vi "ACM RFPM Calibration Verify .vi"() -> ()   [LabVIEW 2023, in "ACM Visa Driver.lvlib"]
uses:
  ACM Visa Driver.lvlib
  API/Controls/ACM Paths.ctl
  API/Controls/ACM Switch States.ctl
  HFNetworkAnalysis/Controls/Unit.ctl
  HFNetworkAnalysis/Controls/Quantity.ctl
  <instrlib>/niRFPM/niRFPM.llb/NI-RFPM Fetch S-Parameter Measurements Complex.vi
  HFNetworkAnalysis/Support VIs/Convert Unit (DBL Array).vi
  HFNetworkAnalysis/NI_HFNetworkAnalysis.lvlib
panel:
  in  "Tab Control":enum32{"Magnitude", "Phase"}(tab)
  out "Magnitude":T1(array[cluster])=[[{"XY Graph"=[{"frequency"=array[531 elements], "yi"=array[531 elements]}, {"frequency"=array[531 elements], "yi"=array[531 elements]}], "String"="S11"}, {"XY Graph"=[{"frequency"=array[531 elements], "yi"=array[531 elements]}, {"frequency"=array[531 elements], "yi"=array[531 elements]}], "String"="S12"}], [{"XY Graph"=[{"frequency"=array[531 elements], "yi"=array[531 elements]}, {"frequency"=array[531 elements], "yi"=array[531 elements]}], "String"="S21"}, {"XY Graph"=[{"frequency"=array[531 elements], "yi"=array[531 elements]}, {"frequency"=array[531 elements], "yi"=array[531 elements]}], "String"="S22"}]]
  out "Phase":T1(array[cluster])=[[{"XY Graph"=[{"frequency"=array[531 elements], "yi"=array[531 elements]}, {"frequency"=array[531 elements], "yi"=array[531 elements]}], "String"="S11"}, {"XY Graph"=[{"frequency"=array[531 elements], "yi"=array[531 elements]}, {"frequency"=array[531 elements], "yi"=array[531 elements]}], "String"="S12"}], [{"XY Graph"=[{"frequency"=array[531 elements], "yi"=array[531 elements]}, {"frequency"=array[531 elements], "yi"=array[531 elements]}], "String"="S21"}, {"XY Graph"=[{"frequency"=array[531 elements], "yi"=array[531 elements]}, {"frequency"=array[531 elements], "yi"=array[531 elements]}], "String"="S22"}]]
  in  "ACM Ports":T2[](array[typedef])=["A", "B"]
  in  "ACM resource name":refnum<visa-resource-name>="USB0::0x2226::0x000F::00000000::INSTR"
  in  "Sweep Setting Name":string="vectorSweep"
  in  "RFPM Ports":string[](array[string])=["port25", "port27"]
  in  "Calibration Storage File Path":path=path "C:/jenkins/workspace/InstallRunCentaurus1910@2/Sales/Semi/projects/RF Calibration/CM ACM VISA Driver/docs/Vulcan_Msmt_VBF-4440/ACM4509_TXecal_RXecal/NI5534_ACM4509_TXecal_RXecal_LowPwr_100HzRBW.tdms"
  out "error out":errorcluster {"code" format="%.0x"}
  in  "Switch":refnum<k15>="VST0" caption="logical name (\"SampleSwitch\")"
  in  "VST":refnum<k15>="VST0"
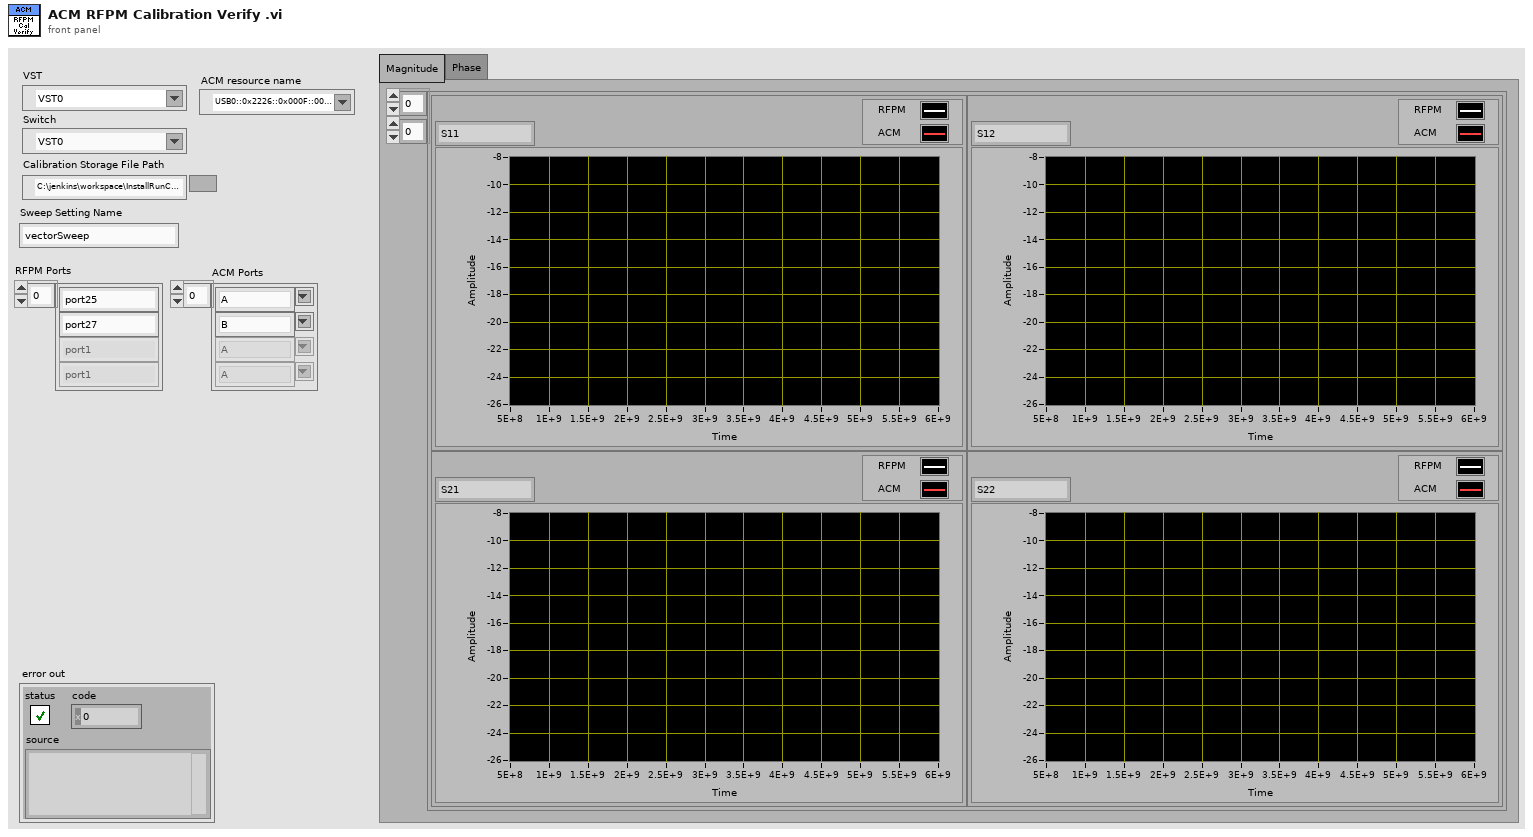
[diagram p1: front panel]
types:
  T1 = cluster{"XY Graph":cluster{"frequency":dbl[], "yi":dbl[]}[], "String":string}[][]
  T2 = typedef "ACM Visa Driver.lvlib/ACM Paths.ctl" = string
  T3 = typedef "ACM Visa Driver.lvlib/ACM Switch States.ctl" = string
  T4 = typedef "NI_HFNetworkAnalysis.lvlib/Unit.ctl" = enum16{"No", "s", "Hz", "V", "A", "Ohm", "W", "dB", "dBV", "dBA", "dBm", "percent", "rad", "deg"}
  T5 = typedef "NI_HFNetworkAnalysis.lvlib/Quantity.ctl" = enum16{"Undefined", "V", "I", "A", "B", "P", "Z", "PowerRatio", "Gamma", "Index"}
  T6 = cluster{"frequency":dbl[], "Converted Data":dbl[]}
  T7 = cluster{"frequency":dbl[], "Converted Data":dbl[]}[]
  T8 = cluster{cluster{"frequency":dbl[], "Converted Data":dbl[]}[], string}
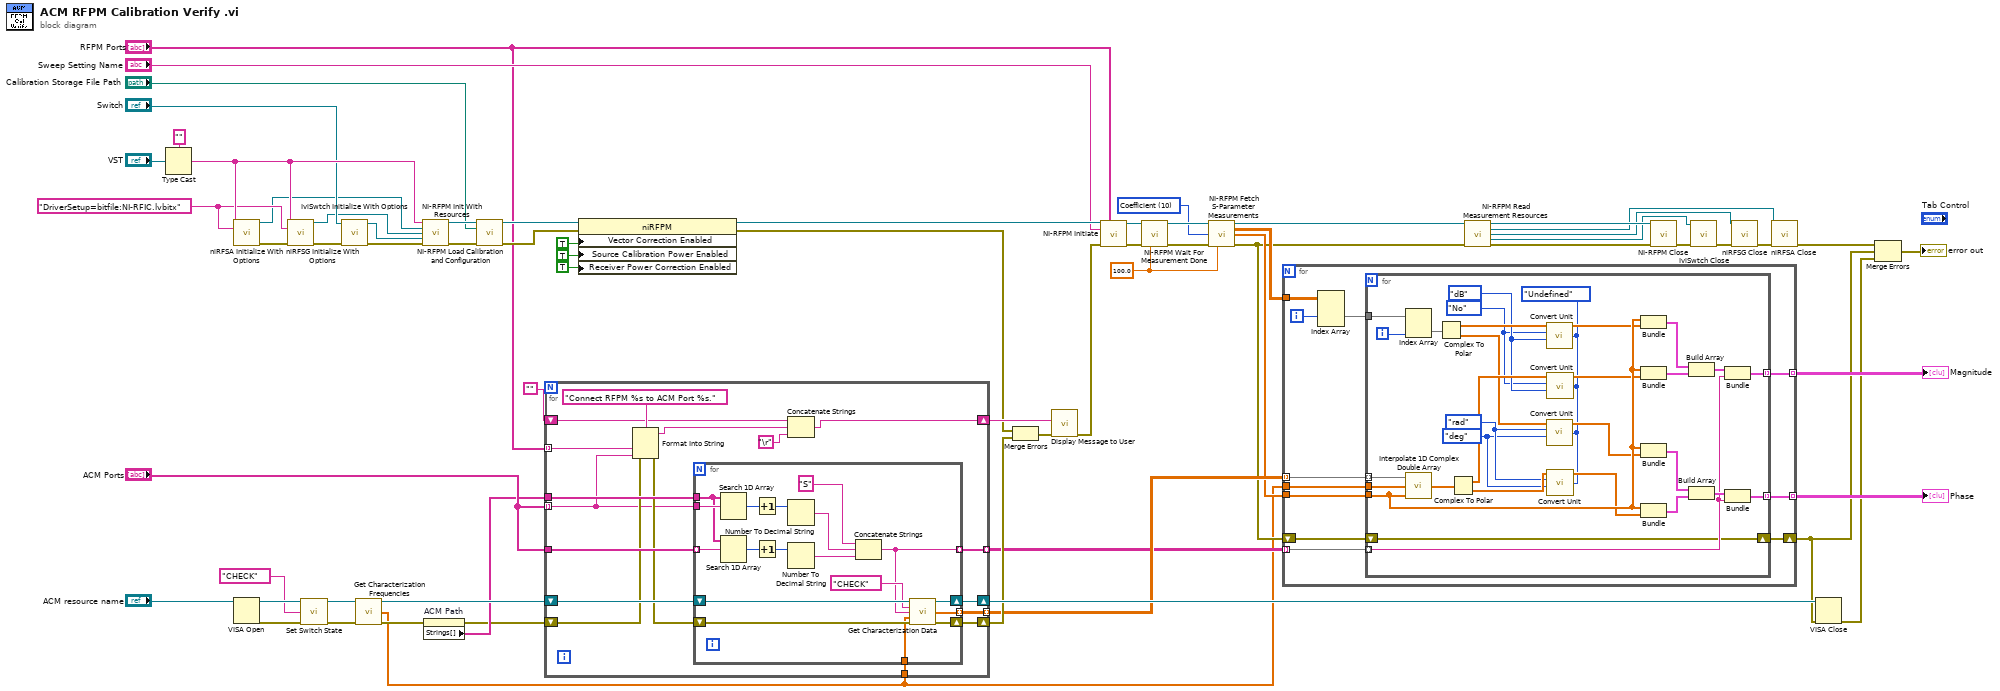
[diagram p0: block diagram]
diagram:
  w54 = 100.0 ("Timeout")
  w53 = 10 items=["Coefficient"=10] ("format")
  w64 = "DriverSetup=bitfile:NI-RFIC.lvbitx"
  n1 = Type Cast(type="", x="VST") -> (*(type *) &x=w65:string)
  n2 = call <instrlib>:"niRFSA Initialize With Options.vi"("resource name"=w65, "option string"=w64) -> ("instrument handle out"=w40:refnum<k15>, "error out"=w44:errorcluster)  [unwired: 12 in]
  n3 = VISA Open(VISA resource name="ACM resource name") -> (VISA resource name=w28:refnum<visa-resource-name>, error out=w30:errorcluster)  [unwired: 4 in]
  n4 = call <instrlib>:"niRFSG Initialize With Options.vi"("resource name"=w65, "option string"=w64, "error in"=w44) -> ("instrument handle"=w41:refnum<k15>, "error out"=w45:errorcluster)  [unwired: 11 in]
  n5 = call "Set Switch State.vi"("VISA resource name"=w28, "Switch State"=T3 "CHECK", "error in (no error)"=w30) -> ("VISA resource name out"=w27:refnum<visa-resource-name>, "error out"=w20:errorcluster)  [unwired: 11 in]
  n6 = call <vilib>:"IviSwtch Initialize With Options.vi"("error in (no error)"=w45, "logical name (\"SampleSwitch\")"="Switch") -> ("error out"=w42:errorcluster, "instrument handle out"=w43:refnum<k15>)  [unwired: 8 in]
  n7 = call "Get Characterization Frequencies.vi"("VISA resource name"=w27, "error in (no error)"=w20) -> ("VISA resource name out"=w29:refnum<visa-resource-name>, "S-Par Characterization Frequencies"=w1:dbl[], "error out"=w24:errorcluster)  [unwired: 11 in]
  n8 = call <instrlib>:"NI-RFPM Init With Resources.vi"("resource name"=w65, "RFSA handle"=w40, "RFSG handle"=w41, "Switch handle"=w43, "error in"=w42) -> ("instrument handle out"=w61:refnum<k15>, "error out"=w58:errorcluster)  [unwired: 9 in]
  n9 = property on="ACM Path" class="CmbBox (strict)"(error in=w24) -> (error out=w22:errorcluster, "Strings[]"=w23:string[])  [unwired: 1 in, 1 out]
  n10 = call <instrlib>:"NI-RFPM Load Calibration and Configuration.vi"("NI-5530 handle in"=w61, "Calibration Storage File Path"="Calibration Storage File Path", "error in"=w58) -> ("instrument handle out"=w60:refnum<k15>, "error out"=w59:errorcluster)  [unwired: 11 in]
  n11 = for {
    tunnel: "ACM Ports" -> [w70] mode=indexing
    tunnel: "ACM Ports" -> [w83]
    tunnel: w23 -> [w82]
    shift-right: [w81] -> w21
    shift-left: w29 -> [w84]
    shift-right: [w80] -> w15
    shift-left: w22 -> [w78]
    tunnel: [w79] -> w12 mode=indexing
    shift-right: [w73] -> w17
    shift-left: "" -> [w75]
    tunnel: "RFPM Ports" -> [w71] mode=indexing
    tunnel: [w69] -> w6 mode=indexing
    tunnel: w1 -> [w68]
    n12 = Format Into String(format string="Connect RFPM %s to ACM Port %s.", error in=w78, w71, w70) -> (resulting string=w74:string, error out=w77:errorcluster)  [unwired: 1 in]
    n13 = for {
      tunnel: w83 -> [w96] mode=indexing
      tunnel: w70 -> [w97]
      tunnel: w82 -> [w95]
      shift-right: [w91] -> w81
      shift-left: w84 -> [w102]
      shift-right: [w92] -> w80
      shift-left: w77 -> [w101]
      tunnel: [w88] -> w79 mode=indexing
      tunnel: [w86] -> w69 mode=indexing
      tunnel: w68 -> [w85]
      n14 = Search 1D Array(1D array=w95, element=w97) -> (index of element=w99:i32)  [unwired: 1 in]
      n15 = Search 1D Array(1D array=w95, element=w96) -> (index of element=w94:i32)  [unwired: 1 in]
      n16 = Increment(x=w99) -> (x+1=w90:i32)
      n17 = Increment(x=w94) -> (x+1=w89:i32)
      n18 = Number To Decimal String(number=w90) -> (decimal integer string=w98:string)  [unwired: 1 in]
      n19 = Number To Decimal String(number=w89) -> (decimal integer string=w93:string)  [unwired: 1 in]
      n20 = Concatenate Strings("S" ("string"), w98, w93) -> (w86:string)
      n21 = call "Get Characterization Data.vi"("VISA resource name"=w102, "ACM Path"=T2 "CHECK", "S-Parameter"=w86, "Characterization Frequencies (for Temp Co)"=w85, "error in (no error)"=w101) -> ("VISA resource name out"=w91:refnum<visa-resource-name>, "S-Par Characterization Data"=w88:cdb[], "error out"=w92:errorcluster)  [unwired: 8 in]
    }
    n22 = Concatenate Strings(w75, w74, "\r") -> (w73:string)
  }
  n23 = property class="niRFPM"(reference=w60, error in=w59, "Vector Correction Enabled"=TRUE ("Measurement:Vector Correction Enabled"), "Source Calibration Power Enabled"=TRUE ("Calibration:Source Power Correction Enabled"), "Receiver Power Correction Enabled"=TRUE ("Calibration:Receiver Power Correction Enabled")) -> (reference out=w57:refnum<k15>, error out=w13:errorcluster)
  n24 = Merge Errors(w13, w15) -> (w14:errorcluster)
  n25 = call "Display Message to User"("error in (no error)"=w14, "Message"=w17) -> ("error out"=w19:errorcluster)  [unwired: 8 in, 1 out]
  n26 = call <instrlib>:"NI-RFPM Initiate.vi"("instrument handle"=w57, "Ports"="RFPM Ports", "Sweep Setting Name"="Sweep Setting Name", "error in"=w19) -> ("instrument handle out"=w52:refnum<k15>, "error out"=w51:errorcluster)  [unwired: 10 in]
  n27 = call <instrlib>:"NI-RFPM Wait For Measurement Done.vi"("instrument handle"=w52, "error in"=w51, "Timeout"=w54) -> ("instrument handle out"=w56:refnum<k15>, "error out"=w55:errorcluster)  [unwired: 11 in]
  n28 = call-poly <instrlib>:"NI-RFPM Fetch S-Parameter Measurements.vi"("instrument handle"=w56, "format"=w53, "error in"=w55, "Timeout"=w54) -> ("instrument handle out"=w62:refnum<k15>, "data"=w11:cdb[][][], "frequency"=w10:dbl[], "error out"=w7:errorcluster)  [unwired: 7 in, 1 out]
  n29 = for {
    tunnel: w12 -> [w111] mode=indexing
    tunnel: w11 -> [w113]
    tunnel: w1 -> [w110]
    tunnel: w10 -> [w109]
    tunnel: [w108] -> w9 mode=indexing
    shift-right: [w106] -> w2
    shift-left: w7 -> [w105]
    tunnel: w6 -> [w104] mode=indexing
    tunnel: [w103] -> w5 mode=indexing
    i -> [w107]
    n30 = Index Array(array=w113, index (dim 1)=w107) -> (element=w112:cdb[][])  [unwired: 2 in]
    n31 = for {
      tunnel: w112 -> [w143]
      tunnel: w111 -> [w142] mode=indexing
      tunnel: w110 -> [w141]
      tunnel: w109 -> [w131]
      tunnel: [w140] -> w108 mode=indexing
      shift-right: [w127] -> w106
      shift-left: w105 -> [w127]
      tunnel: w104 -> [w130] mode=indexing
      tunnel: [w132] -> w103 mode=indexing
      i -> [w136]
      w115 = Unit."deg" ("Base Unit")
      w116 = Unit."rad" ("Target Unit")
      w114 = Quantity."Undefined" ("Quantity")
      w121 = Unit."No" ("Base Unit")
      w123 = Unit."dB" ("Target Unit")
      n32 = Index Array(array=w143, index (col)=w136) -> (element=w128:cdb[])  [unwired: 1 in]
      n33 = call "Interpolate 1D Complex Double Array.vi"("xi"=w131, "X"=w141, "Y"=w142) -> ("yi"=w129:cdb[])
      n34 = Complex To Polar(r * e^(i*theta)=w128) -> (r=w125:dbl[], theta=w117:dbl[])
      n35 = Complex To Polar(r * e^(i*theta)=w129) -> (r=w124:dbl[], theta=w120:dbl[])
      n36 = call-poly "Convert Unit.vi"("Quantity"=w114, "Target Unit"=w123, "Base Unit"=w121, "Data"=w125) -> ("Converted Data"=w126:dbl[])  [unwired: 3 in, 1 out]
      n37 = call-poly "Convert Unit.vi"("Quantity"=w114, "Target Unit"=w115, "Base Unit"=w116, "Data"=w117) -> ("Converted Data"=w118:dbl[])  [unwired: 3 in, 1 out]
      n38 = call-poly "Convert Unit.vi"("Quantity"=w114, "Target Unit"=w123, "Base Unit"=w121, "Data"=w124) -> ("Converted Data"=w122:dbl[])  [unwired: 3 in, 1 out]
      n39 = call-poly "Convert Unit.vi"("Quantity"=w114, "Target Unit"=w115, "Base Unit"=w116, "Data"=w120) -> ("Converted Data"=w119:dbl[])  [unwired: 3 in, 1 out]
      n40 = Bundle("frequency"=w131, "Converted Data"=w126) -> (w139:T6)  [unwired: 1 in]
      n41 = Bundle("frequency"=w131, "Converted Data"=w122) -> (w138:T6)  [unwired: 1 in]
      n42 = Bundle("frequency"=w131, "Converted Data"=w118) -> (w133:T6)  [unwired: 1 in]
      n43 = Bundle("frequency"=w131, "Converted Data"=w119) -> (w134:T6)  [unwired: 1 in]
      n44 = Build Array(w139, w138) -> (w137:T7)
      n45 = Build Array(w133, w134) -> (w135:T7)
      n46 = Bundle(w137, w130) -> (w140:T8)  [unwired: 1 in]
      n47 = Bundle(w135, w130) -> (w132:T8)  [unwired: 1 in]
    }
  }
  "Magnitude" <- w9
  "Phase" <- w5
  n48 = call <instrlib>:"NI-RFPM Read Measurement Resources.vi"("NI-5530 handle in"=w62, "error in"=w7) -> ("NI-5530 handle out"=w39:refnum<k15>, "RFSA handle"=w33:refnum<k15>, "RFSG handle"=w34:refnum<k15>, "Switch handle"=w35:refnum<k15>, "error out"=w32:errorcluster)  [unwired: 9 in]
  n49 = call <instrlib>:"NI-RFPM Close.vi"("NI-5530 handle in"=w39, "error in"=w32) -> ("error out"=w38:errorcluster)  [unwired: 13 in]
  n50 = call <vilib>:"IviSwtch Close.vi"("error in (no error)"=w38, "instrument handle"=w35) -> ("error out"=w37:errorcluster)  [unwired: 9 in]
  n51 = call <instrlib>:"niRFSG Close.vi"("instrument handle"=w34, "error in"=w37) -> ("error out"=w36:errorcluster)  [unwired: 13 in]
  n52 = call <instrlib>:"niRFSA Close.vi"("instrument handle"=w33, "error in"=w36) -> ("error out"=w4:errorcluster)  [unwired: 13 in]
  n53 = VISA Close(VISA resource name=w21, error in (no error)=w2) -> (error out=w3:errorcluster)
  n54 = Merge Errors(w4, w2, w3) -> (→"error out":errorcluster)
